vi "Create Evaluations.vi"(8 "error in (no error)":errorcluster, 11 "IEvaluation in":refnum<class "LTE_OBW.lvclass">) -> (0 "error out":errorcluster, 2 "Evaluations Out":T1[](array[typedef]) {"Low Limit" format="%#_13g"; "SI Scaling" items=["femto"=-15, "pico"=-12, "nano"=-9, "micro"=-6, "milli"=-3, "percent"=-2, ""=0, "kilo"=3, "mega"=6, "giga"=9, "tera"=12]}, 3 "IEvaluation out":refnum<class "LTE_OBW.lvclass">)   [LabVIEW 2016, in "SeqAuto Evaluations.lvlib" / "LTE_OBW.lvclass"]
uses:
  LTE_OBW.lvclass
  C:/STS/Common/1.0/Sequence Automation/Plugins/SeqAuto IEvaluation.lvlibp/SeqAuto IEvaluation.lvclass
  Plugins/TestStand API Tools (TSAT).lvlibp/Evaluation Actions/Includes/Controls/TSAT Evaluation.ctl
  Plugins/TestStand API Tools (TSAT).lvlibp/Evaluation Actions/Includes/Controls/TSAT Eval SI Unit Scaling.ctl
  Plugins/TestStand API Tools (TSAT).lvlibp/Evaluation Actions/Includes/Controls/TSAT Evaluation Type.ctl
  LTE_OBW.lvclass/LTE_OBW.ctl
  Read SA Pin.vi
  Plugins/SeqAuto IEvaluation.lvlibp/Read Measurement Name.vi
  Plugins/TestStand API Tools (TSAT).lvlibp/Evaluation Actions/TSAT Evaluation Actions.lvlib
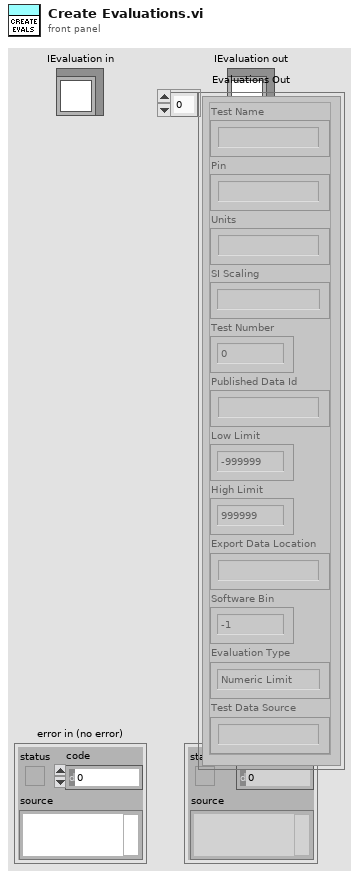
[diagram p1: front panel]
types:
  T1 = typedef "TestStand API Tools (TSAT).lvlibp/TSAT Evaluation Actions.lvlib/TSAT Evaluation.ctl" = cluster{"Test Name":string, "Pin":string, "Units":string, "SI Scaling":T2, "Test Number":i32, "Published Data Id":string, "Low Limit":dbl, "High Limit":dbl, "Export Data Location":string, "Software Bin":i64, "Evaluation Type":T3, "Test Data Source":string}
  T2 = typedef "TestStand API Tools (TSAT).lvlibp/TSAT Evaluation Actions.lvlib/TSAT Eval SI Unit Scaling.ctl" = i16
  T3 = typedef "TestStand API Tools (TSAT).lvlibp/TSAT Evaluation Actions.lvlib/TSAT Evaluation Type.ctl" = enum16{"Numeric Limit", "Pass/Fail", "None"}
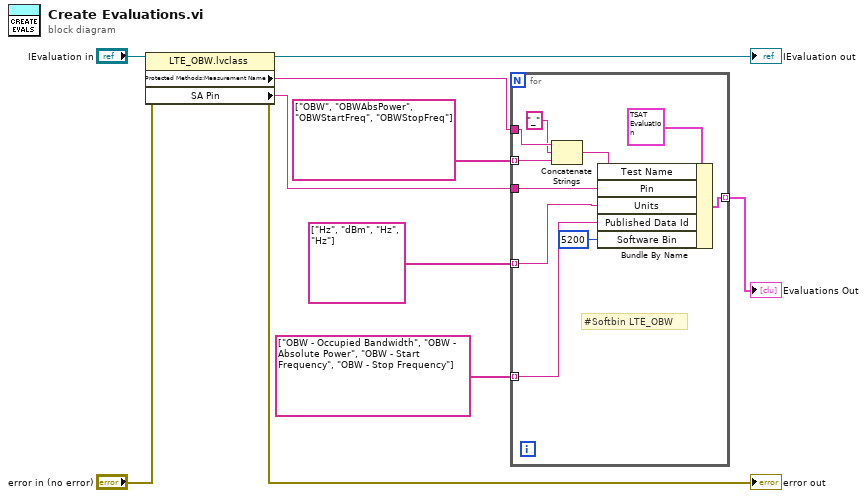
[diagram p0: block diagram]
diagram:
  n1 = property class="LTE_OBW.lvclass"(reference="IEvaluation in", error in="error in (no error)") -> (reference out=→"IEvaluation out":refnum<class "LTE_OBW.lvclass">, error out=→"error out":errorcluster, "Protected Methods:Measurement Name"=w4:string, "SA Pin"=w5:string)
  n2 = for {
    tunnel: [w19] -> w6 mode=indexing
    tunnel: w5 -> [w18]
    tunnel: w4 -> [w17]
    tunnel: string[] ["OBW", "OBWAbsPower", "OBWStartFreq", "OBWStopFreq"] -> [w16] mode=indexing
    tunnel: string[] ["Hz", "dBm", "Hz", "Hz"] -> [w13] mode=indexing
    tunnel: string[] ["OBW - Occupied Bandwidth", "OBW - Absolute Power", "OBW - Start Frequency", "OBW - Stop Frequency"] ("Array") -> [w12] mode=indexing
    # "#Softbin LTE_OBW"
    n3 = Concatenate Strings(w17, "_" ("string"), w16) -> (w15:string)
    n4 = Bundle By Name(cluster=T1 {"Test Name"="", "Pin"="", "Units"="", "SI Scaling"=0, "Test Number"=0, "Published Data Id"="", "Low Limit"=-999999.0, "High Limit"=999999.0, "Export Data Location"="", "Software Bin"=-1, "Evaluation Type"=enum."Numeric Limit", "Test Data Source"=""} ("Evaluation"), "Test Name"=w15, "Pin"=w18, "Units"=w13, "Published Data Id"=w12, "Software Bin"=i64 5200) -> (w19:T1)
  }
  "Evaluations Out" <- w6
